vi "Get Scan Subanel Values.vi"(8 "error in (no error)":errorcluster, 11 "Scan SBlock in":refnum<class "Scan SBlock.lvclass">) -> (0 "error out":errorcluster, 2 "No. of steps":u32, 3 "Scan SBlock out":refnum<class "Scan SBlock.lvclass">, 4 "Array of Parameters":T1[](array[typedef]), 5 "Array from List":T3[](array[typedef]))   [LabVIEW 2020, in "Run Utilities.lvlib" / "Scan SBlock.lvclass"]
uses:
  Scan SBlock.lvclass
  Advanced Parameters - list.ctl
  Advanced Parameters.ctl
  Advanced Panel Parameter Mode.ctl
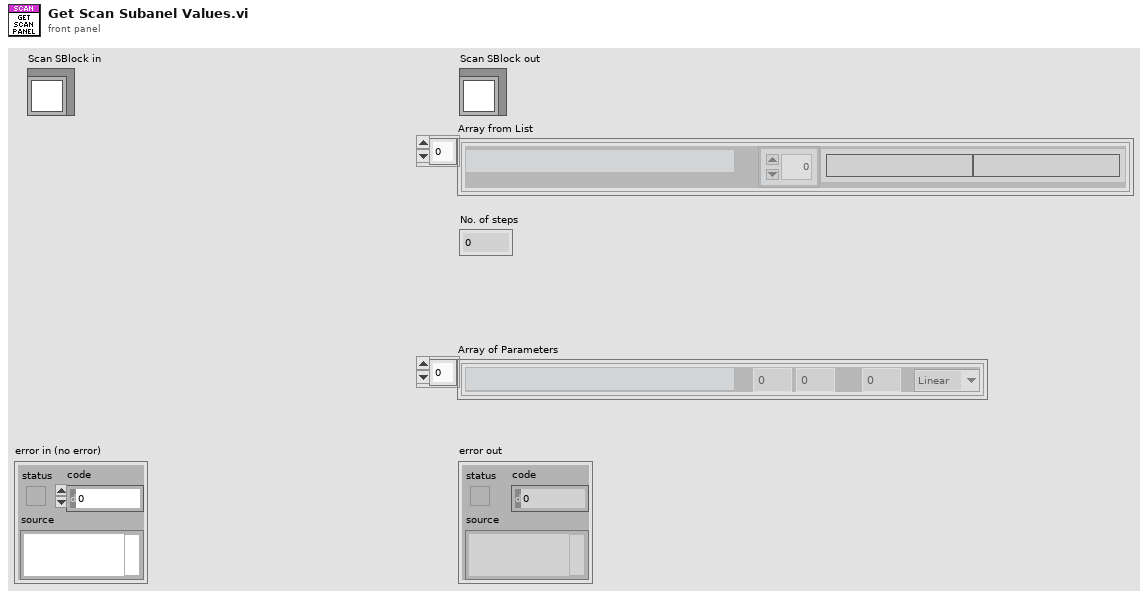
[diagram p1: front panel]
types:
  T1 = typedef "Run Utilities.lvlib/Scan SBlock.lvclass/Advanced Parameters.ctl" = cluster{"Param":string, "From":dbl, "To":dbl, "Step":dbl, "Mode":T2}
  T2 = typedef "Run Utilities.lvlib/Scan SBlock.lvclass/Advanced Panel Parameter Mode.ctl" = enum16{"Linear", "Log", "LINKED"}
  T3 = typedef "Run Utilities.lvlib/Scan SBlock.lvclass/Advanced Parameters - list.ctl" = cluster{"Param":string, "List of values":string[]}
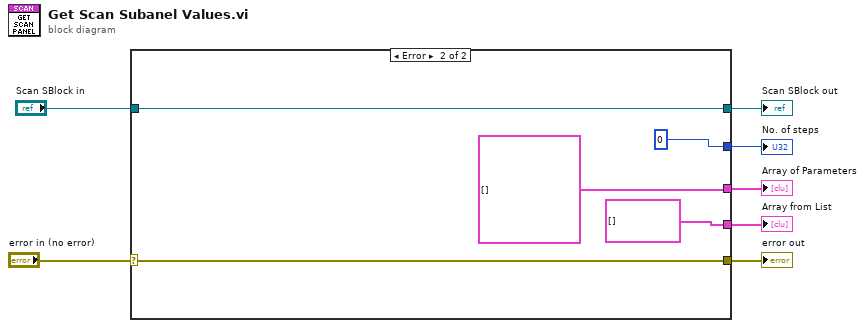
[diagram p0: block diagram]
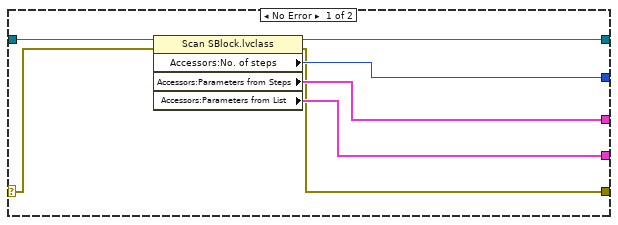
[diagram p2: hidden frame]
diagram:
  n1 = case shown="Error" "error in (no error)" {
    selector: "error in (no error)" -> [w9 w19]
    tunnel: [w8 w19] -> w6
    tunnel: [w13 w18] -> w2
    tunnel: "Scan SBlock in" -> [w14 w18]
    tunnel: [w10 u32 0 ("No. of steps")] -> w5
    tunnel: [w12 T3[] [] ("Array from List")] -> w4
    tunnel: [w11 T1[] [] ("Array of Parameters")] -> w3
    frame No Error {
      n2 = property class="Scan SBlock.lvclass"(reference=w14, error in=w9) -> (reference out=w13:refnum<class "Scan SBlock.lvclass">, error out=w8:errorcluster, "Accessors:No. of steps"=w10:u32, "Accessors:Parameters from Steps"=w11:T1[], "Accessors:Parameters from List"=w12:T3[])
    }
    frame Error {
    }
  }
  "error out" <- w6
  "No. of steps" <- w5
  "Array from List" <- w4
  "Array of Parameters" <- w3
  "Scan SBlock out" <- w2
